vi "Helper Action.vi"(8 "error in (no error)":errorcluster, 9 "Message Data":variant, 10 "Message":string, 11 "Customer With Phone In":refnum<class "Customer With Phone.lvclass">) -> (0 "error out":errorcluster, 1 "Exit?":bool, 2 "Loop Period [ms]":u32=1000, 3 "Customer With Phone Out":refnum<class "Customer With Phone.lvclass">)   [LabVIEW 2020, in "Customer With Phone.lvclass"]
doc: "The specific action implemented in the helper loop. Multiple different actions may be supported by using the Message and Message Data input to separate them. Any number of helper loops may run in parallell running the same or different actions. \nThe helper loop rate is controlled by the Loop Perid output of this method. \nIf this method throws an error, the helper loop will stop. The error will be sent to the error handler configured for the process. To stop it intentionally, the Stop Helper Loop.vi should be used. \nOne caveat with the helper loop is that it will have a copy of the object attributes as they were when the helper loop was started. If the attributes are updated, the helper loop will need to be restarted to refresh attributes."
uses:
  Customer With Phone.lvclass
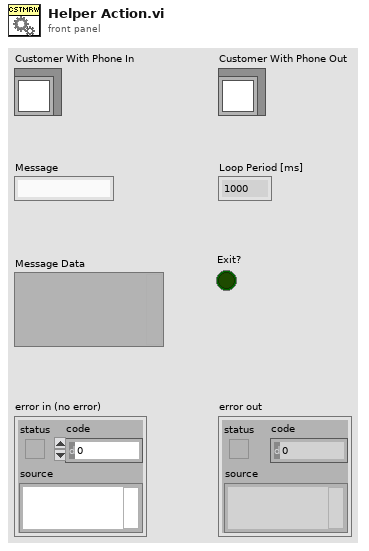
[diagram p1: front panel]
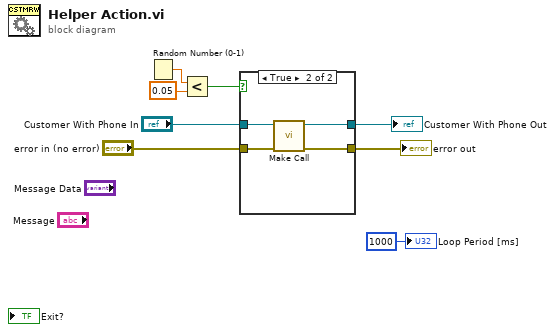
[diagram p0: block diagram]
diagram:
  n1 = Random Number (0-1)() -> (number: 0 to 1=w7:dbl)
  n2 = Less?(x=w7, y=0.05) -> (x < y?=w4:bool)
  n3 = case shown="True" w4 {
    tunnel: "Customer With Phone In" -> [w10 w14]
    tunnel: [w10 w13] -> w5
    tunnel: "error in (no error)" -> [w9 w12]
    tunnel: [w9 w11] -> w2
    frame False {
    }
    frame True {
      n4 = call "Make Call.vi"("error in (no error)"=w12, "Customer With Phone In"=w14) -> ("error out"=w11:errorcluster, "Customer With Phone Out"=w13:refnum<class "Customer With Phone.lvclass">)  [unwired: 8 in]
    }
  }
  "error out" <- w2
  "Customer With Phone Out" <- w5
  "Loop Period [ms]" <- u32 1000 ("Loop Period [ms]")
